vi "FIFO Check.vi"(0 "FPGA Ref in":T3, 5 "Read at least # points":u32, 7 "Imaging Protocol":T1, 11 "error in (no error)":errorcluster) -> (4 "FPGA Ref out":T3, 6 "Elements Available":T2, 8 "Both channels no more data (delayed by 1 iteration)":bool, 10 "Data available or data has just completed (read the FIFO)":bool, 15 "error out":errorcluster)   [LabVIEW 2017]
uses:
  RIG-SPECIFIC FILES/FPGA Refs/FPGA Ref.ctl
  Acquisition/Typedefs/FIFO elements available.ctl
  Typedefs/Imaging Protocols enum.ctl
  <vilib>/Utility/error.llb/Error Cluster From Error Code.vi
  <vilib>/rvi/errors/niLvFpgaAdjustHostInterfaceError.vi
  <vilib>/rvi/interface/nirviMethod/nirviMethod.xnode
  <vilib>/rvi/errors/niLvFpgaMergeErrorWithErrorCode.vi
  <vilib>/FPGAPlugInAG/Dynamic/niLvFpga_ReadFifo_Dynamic.vi
panel:
  out "No more data Ch1":bool
  out "No more data Ch0":bool
  out "Registered peak value":dbl
  in  "Timeout (ms)":i32=30
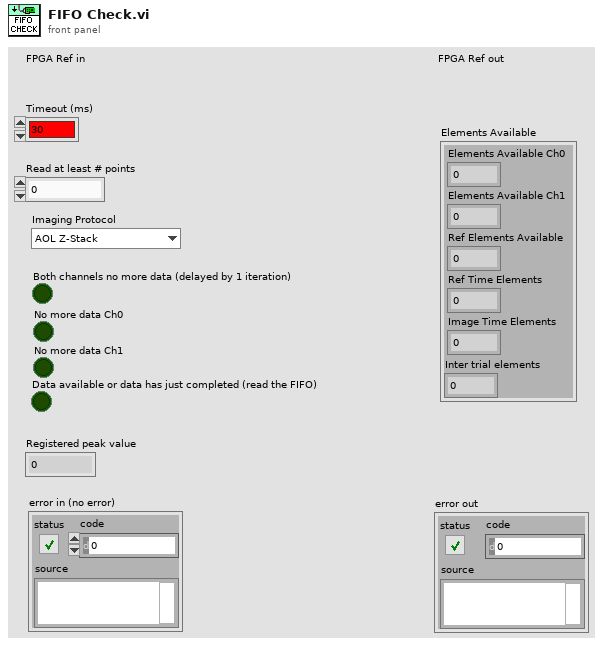
[diagram p1: front panel]
types:
  T1 = typedef "Imaging Protocols enum.ctl" = enum16{"AOL Z-Stack", "Motor Z Stack", "Functional Acquisition", "Single Plane Acquisition", "Volume Acquisition", "Live Imaging", "Live Plane Imaging", "Live Volume Imaging"}
  T2 = typedef "FIFO elements available.ctl" = cluster{"Elements Available Ch0":u32, "Elements Available Ch1":u32, "Ref Elements Available":u32, "Ref Time Elements":u32, "Image Time Elements":u32, "Inter trial elements":u32}
  T3 = typedef "FPGA Ref.ctl" = refnum<k20>
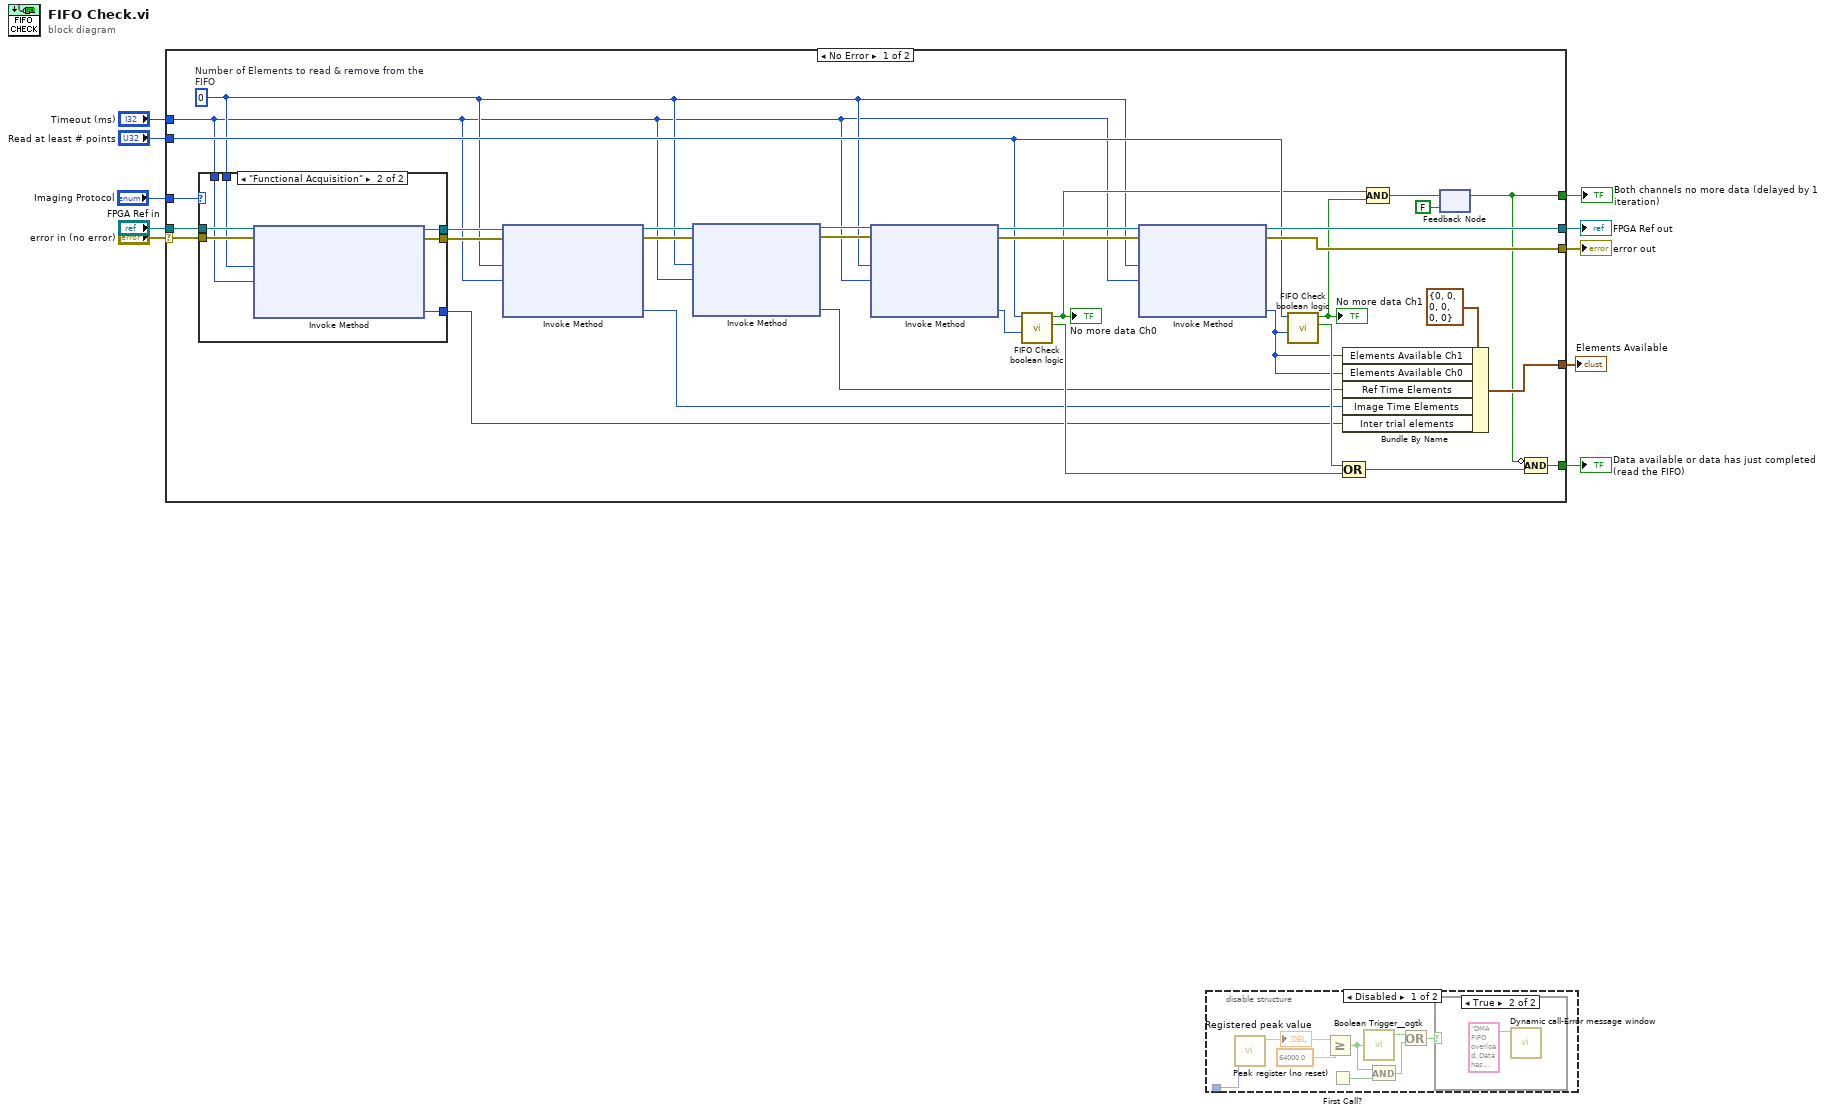
[diagram p0: block diagram]
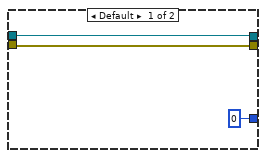
[diagram p2: hidden frame]
diagram:
  n1 = case shown="No Error" "error in (no error)" {
    selector: "error in (no error)" -> [w17 w54]
    tunnel: [w27 _] -> w10
    tunnel: [w42 w53] -> w9
    tunnel: "FPGA Ref in" -> [w18 w53]
    tunnel: "Timeout (ms)" -> [w13 _]
    tunnel: [w39 w54] -> w6
    tunnel: "Read at least # points" -> [w38 _]
    tunnel: [w36 _] -> w2
    tunnel: [w26 _] -> w3
    tunnel: "Imaging Protocol" -> [w11 _]
    frame No Error {
      w14 = u32 0  # Number of Elements to read & remove from the FIFO
      n2 = case shown="\"Functional Acquisition\"" w11 {
        tunnel: w18 -> [w45 w52]
        tunnel: w17 -> [w44 w51]
        tunnel: [w45 w50] -> w16
        tunnel: [w44 w49] -> w15
        tunnel: w14 -> [_ w48]
        tunnel: w13 -> [_ w47]
        tunnel: [u32 0 ("Elements Remaining") w46] -> w12
        frame Default {
        }
        frame "Functional Acquisition" {
          n3 = xnode ("Invoke Method")("FPGA VI Reference In"=w52, "error in"=w51, "Number of Elements"=w48, "Timeout (ms)"=w47) -> ("FPGA VI Reference Out"=w50:T3, "error out"=w49:errorcluster, "Elements Remaining"=w46:u32)  [unwired: 1 out]
        }
      }
      n4 = xnode ("Invoke Method")("FPGA VI Reference In"=w16, "error in"=w15, "Number of Elements"=w14, "Timeout (ms)"=w13) -> ("FPGA VI Reference Out"=w22:T3, "error out"=w21:errorcluster, "Elements Remaining"=w19:u32)  [unwired: 1 out]
      n5 = xnode ("Invoke Method")("FPGA VI Reference In"=w22, "error in"=w21, "Number of Elements"=w14, "Timeout (ms)"=w13) -> ("FPGA VI Reference Out"=w25:T3, "error out"=w24:errorcluster, "Elements Remaining"=w23:u32)  [unwired: 1 out]
      n6 = xnode ("Invoke Method")("FPGA VI Reference In"=w25, "error in"=w24, "Number of Elements"=w14, "Timeout (ms)"=w13) -> ("FPGA VI Reference Out"=w41:T3, "error out"=w40:errorcluster, "Elements Remaining"=w34:u32)  [unwired: 1 out]
      n7 = call "FIFO Check boolean logic.vi"("Elements Remaining"=w34, "Read at least"=w38) -> ("Read FIFO"=w35:bool, "No more data"=w32:bool)  [unwired: 8 in]
      "No more data Ch0" <- w32
      n8 = xnode ("Invoke Method")("FPGA VI Reference In"=w41, "error in"=w40, "Number of Elements"=w14, "Timeout (ms)"=w13) -> ("FPGA VI Reference Out"=w42:T3, "error out"=w39:errorcluster, "Elements Remaining"=w33:u32)  [unwired: 1 out]
      n9 = call "FIFO Check boolean logic.vi"("Elements Remaining"=w33, "Read at least"=w38) -> ("Read FIFO"=w37:bool, "No more data"=w31:bool)  [unwired: 8 in]
      "No more data Ch1" <- w31
      n10 = Bundle By Name(cluster=T2 {"Elements Available Ch0"=0, "Elements Available Ch1"=0, "Ref Elements Available"=0, "Ref Time Elements"=0, "Image Time Elements"=0, "Inter trial elements"=0} ("Elements Available 2"), "Elements Available Ch1"=w33, "Elements Available Ch0"=w33, "Ref Time Elements"=w23, "Image Time Elements"=w19, "Inter trial elements"=w12) -> (w36:T2)
      n11 = Compound Arithmetic op=OR(w37, w35) -> (w28:bool)
      n12 = Compound Arithmetic op=AND(w32, w31) -> (w30:bool)
      n13 = feedback-in #1(w30) -> ()
      n14 = feedback #1(FALSE) -> (w26:bool)
      n15 = Compound Arithmetic op=AND(invert w26, w28) -> (w27:bool)
    }
    frame Error {
    }
  }
  "error out" <- w6
  "FPGA Ref out" <- w9
  "Data available or data has just completed (read the FIFO)" <- w10
  "Both channels no more data (delayed by 1 iteration)" <- w3
  "Elements Available" <- w2
  n16 = disable-structure "Diagram Disable Structure" shown="Disabled" {
    disable-tunnel: _ -> [w62 _]
    frame Disabled {
      n17 = call <userlib>:"Peak register (no reset).vi"("Value in"=w62) -> ("Registered peak value"=w61:dbl)  [unwired: 10 in]
      "Registered peak value" <- w61
      n18 = Greater Or Equal?(x=w61, y=64000.0) -> (x >= y?=w59:bool)
      n19 = First Call?() -> (First Call?: T/F=w58:bool)
      n20 = call <userlib>:"Boolean Trigger__ogtk.vi"("Boolean Input"=w59) -> ("Rising Edge"=w57:bool)  [unwired: 1 in, 1 out]
      n21 = And(x=w59, y=w58) -> (x .and. y?=w56:bool)
      n22 = Or(x=w57, y=w56) -> (x .or. y?=w55:bool)
      n23 = case shown="True" w55 {
        frame False {
        }
        frame True {
          n24 = call "Dynamic call-Error message window.vi"("Error Message"="DMA FIFO overload. Data has been lost.") -> ()  [unwired: 10 in, 1 out]
        }
      }
    }
    frame Enabled {
    }
  }
